vi "Write IV Settings.vi"(8 "error in (no error)":errorcluster, 10 "IV Settings":T1, 11 "Dot Settings in":refnum<class "Dot Settings.lvclass">) -> (0 "error out":errorcluster, 3 "Dot Settings out":refnum<class "Dot Settings.lvclass">)   [LabVIEW 2019, in "Dot Settings.lvclass"]
uses:
  Dot Settings.lvclass
  TypeDefs/IV Settings.ctl
  Dot Settings.lvclass/Dot Settings.ctl
  453b4698-bccb-48d0-a7df-54920c8bac9f.vi
  <vilib>/JDP Science/JSONtext/Variant to JSON Text.vi
  <vilib>/JDP Science/JSONtext/LVClass Serializer/JSONtext LVClass Serializer.lvclass
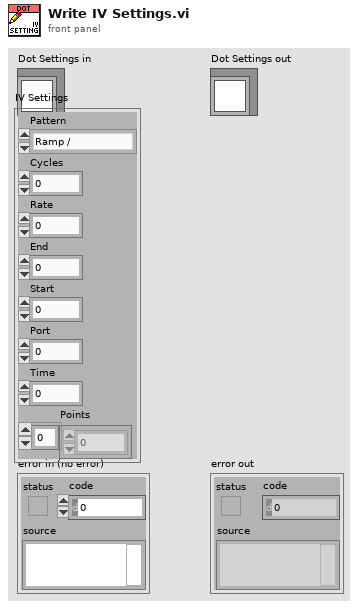
[diagram p1: front panel]
types:
  T1 = typedef "Dot Settings.lvclass/IV Settings.ctl" = cluster{"Pattern":enum16{"Ramp /", "Ramp /\\", "Smooth Ramp _/", "Smooth Ramp _/\\_", "Frequency"}, "Cycles":i32, "Rate":dbl, "End":dbl, "Start":dbl, "Port":u32, "Time":dbl, "Points":dbl[]}
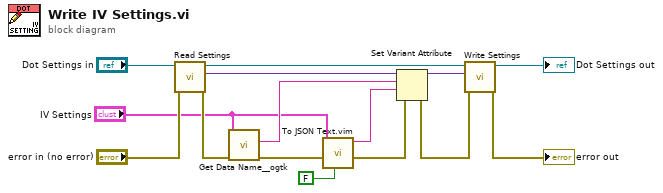
[diagram p0: block diagram]
diagram:
  n1 = call "Read Settings.vi"("error in (no error)"="error in (no error)", "Dot Settings in"="Dot Settings in") -> ("error out"=w9:errorcluster, "Settings"=w12:variant, "Dot Settings out"=w11:refnum<class "Dot Settings.lvclass">)  [unwired: 7 in]
  n2 = call <userlib>:"Get Data Name__ogtk.vi"("error in (no error)"=w9, "Data"="IV Settings") -> ("error out"=w5:errorcluster, "Data Name"=w13:string)  [unwired: 7 in, 1 out]
  n3 = call "To JSON Text.vim"("Pretty Print?"=FALSE, "error in (no error)"=w5, "Anything"="IV Settings") -> ("error out"=w4:errorcluster, "<JSON>"=w2:string)  [unwired: 7 in]
  n4 = Set Variant Attribute(Variant=w12, name=w13, value=w2, error in=w4) -> (Variant out=w10:variant, error out=w8:errorcluster)  [unwired: 1 out]
  n5 = call "Write Settings.vi"("error in (no error)"=w8, "Settings"=w10, "Dot Settings in"=w11) -> ("error out"=→"error out":errorcluster, "Dot Settings out"=→"Dot Settings out":refnum<class "Dot Settings.lvclass">)  [unwired: 7 in]
